vi "TestingImagesRefs.vi"() -> ()   [LabVIEW 2013]
uses:
  <vilib>/vision/Image Controls.llb/IMAQ Image.ctl
panel:
  out "Image 4":T1(plugin-control)
  out "Image 3":T1
  out "Image 2":T1
  out "Image":T1(plugin-control)
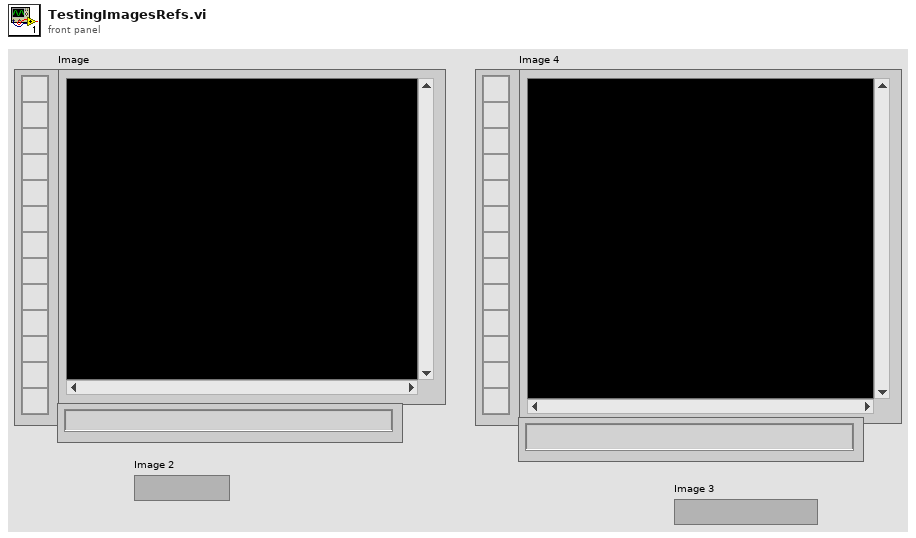
[diagram p1: front panel]
types:
  T1 = typedef "IMAQ Image.ctl" = refnum<image>
  T2 = typedef "Image Type" = u32
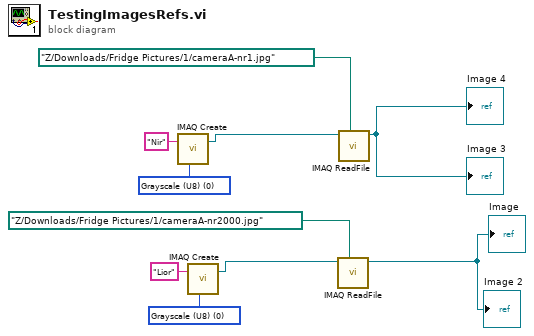
[diagram p0: block diagram]
diagram:
  w8 = T2 0 items=["Grayscale (U8)", "Grayscale (I16)", "Grayscale (SGL)", "Complex (CSG)", "RGB (U32)", "HSL (U32)", "RGB (U64)", "Grayscale (U16)"] ("Image Type")
  w10 = T2 0 items=["Grayscale (U8)", "Grayscale (I16)", "Grayscale (SGL)", "Complex (CSG)", "RGB (U32)", "HSL (U32)", "RGB (U64)", "Grayscale (U16)"] ("Image Type")
  n1 = call "IMAQ Create"("Image Name"="Nir", "Image Type"=w10) -> ("New Image"=w9:T1)  [unwired: 2 in, 2 out]
  n2 = call "IMAQ Create"("Image Name"="Lior", "Image Type"=w8) -> ("New Image"=w7:T1)  [unwired: 2 in, 2 out]
  n3 = call "IMAQ ReadFile"("File Path"=path "Z:/Downloads/Fridge Pictures/1/cameraA-nr2000.jpg" ("Path"), "Image"=w7) -> ("Image Out"=→"Image" →"Image 2":T1)  [unwired: 3 in, 6 out]
  n4 = call "IMAQ ReadFile"("File Path"=path "Z:/Downloads/Fridge Pictures/1/cameraA-nr1.jpg" ("Path"), "Image"=w9) -> ("Image Out"=→"Image 3" →"Image 4":T1)  [unwired: 3 in, 6 out]
